vi "Keithley24XX_measure_snap.vi"() -> ()   [LabVIEW 2018]
uses:
  <instrlib>/Keithley 24XX/Public/Data/Read (Single Point).vi
  <instrlib>/Keithley 24XX/Keithley 24XX.lvlib
panel:
  out "output cluster":T1
  out "error out 2":errorcluster
  out "VISA resource name out":refnum<visa-resource-name>
  in  "error in (no error)":errorcluster
  in  "VISA resource name":refnum<visa-resource-name>
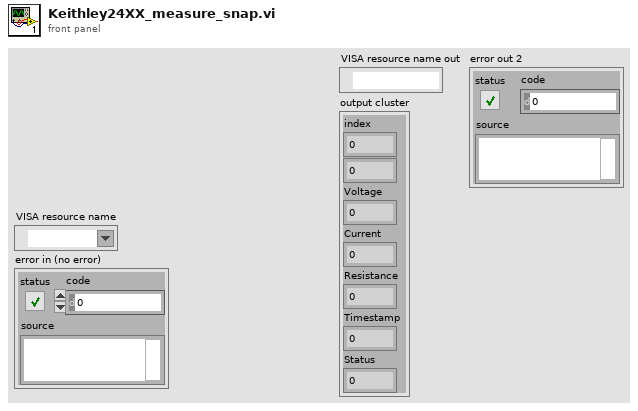
[diagram p1: front panel]
types:
  T1 = cluster{"index":i32, dbl, "Voltage":sgl, "Current":sgl, "Resistance":sgl, "Timestamp":sgl, "Status":sgl}
  T2 = cluster{"Source Mode":enum16{"Voltage", "Current"}, "Source Amplitude":dbl, "Timestamp":sgl, "Status":sgl, "Current":sgl, "Voltage":sgl, "Resistance":sgl}
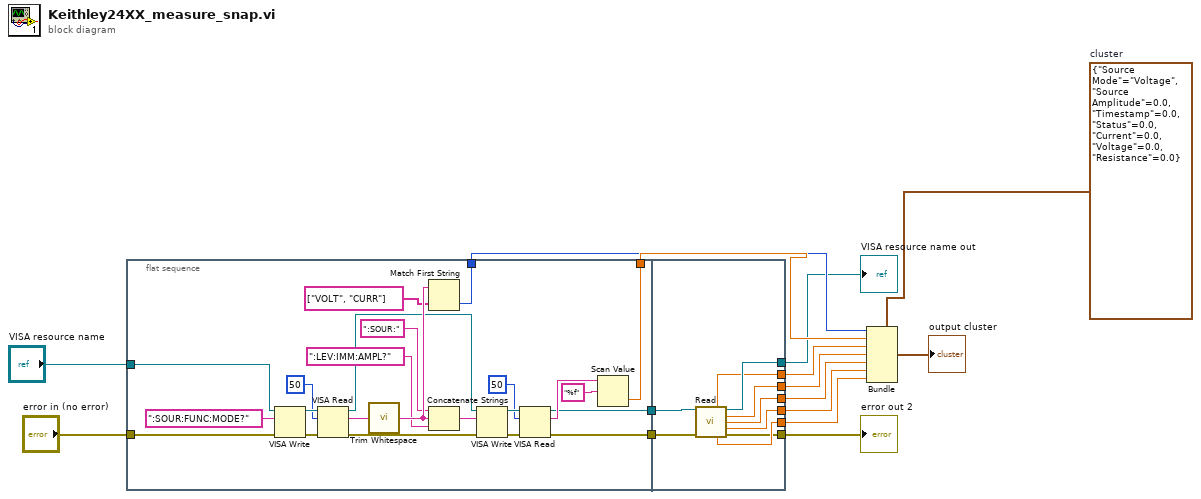
[diagram p0: block diagram]
diagram:
  w1 = T2 {"Source Mode"=enum."Voltage", "Source Amplitude"=0.0, "Timestamp"=0.0, "Status"=0.0, "Current"=0.0, "Voltage"=0.0, "Resistance"=0.0}  # cluster
  n1 = flat-sequence {
    tunnel: "VISA resource name" -> [w19]
    tunnel: "error in (no error)" -> [w18]
    tunnel: [w20] -> w13
    tunnel: [w21] -> w12
    tunnel: [w17] -> w11
    tunnel: [w16] -> w10
    tunnel: [w43] -> w3
    tunnel: [w44] -> w6
    tunnel: w11 -> [w47]
    tunnel: w10 -> [w46]
    tunnel: [w45] -> w9
    tunnel: [w42] -> w8
    tunnel: [w41] -> w7
    tunnel: [w40] -> w5
    tunnel: [w39] -> w4
    frame #0 {
      n2 = VISA Write(VISA resource name=w19, write buffer=":SOUR:FUNC:MODE?", error in (no error)=w18) -> (VISA resource name out=w30:refnum<visa-resource-name>, error out=w29:errorcluster)  [unwired: 1 out]
      n3 = VISA Read(VISA resource name=w30, byte count=u32 50, error in (no error)=w29) -> (VISA resource name out=w34:refnum<visa-resource-name>, read buffer=w37:string, error out=w33:errorcluster)  [unwired: 1 out]
      n4 = call <vilib>:"Trim Whitespace.vi"("string"=w37) -> ("trimmed string"=w38:string)  [unwired: 1 in]
      n5 = Match First String(2:string[] ["VOLT", "CURR"] ("string array"), 3:w38) -> (0:w21:i32)  [unwired: 1 out]
      n6 = Concatenate Strings(":SOUR:" ("string"), w38, ":LEV:IMM:AMPL?" ("string")) -> (w35:string)
      n7 = VISA Write(VISA resource name=w34, write buffer=w35, error in (no error)=w33) -> (VISA resource name out=w32:refnum<visa-resource-name>, error out=w31:errorcluster)  [unwired: 1 out]
      n8 = VISA Read(VISA resource name=w32, byte count=u32 50, error in (no error)=w31) -> (VISA resource name out=w17:refnum<visa-resource-name>, read buffer=w36:string, error out=w16:errorcluster)  [unwired: 1 out]
      n9 = Scan Value(string=w36, format string="%f") -> (value=w20:dbl)  [unwired: 1 in, 1 out]
    }
    frame #1 {
      n10 = call-poly <instrlib>:"Read.vi"("VISA resource name"=w47, "error in (no error)"=w46) -> ("Voltage"=w41:sgl, "VISA resource name out"=w45:refnum<visa-resource-name>, "Current"=w44:sgl, "Resistance"=w40:sgl, "Timestamp"=w39:sgl, "Status"=w43:sgl, "error out"=w42:errorcluster)  [unwired: 7 in]
    }
  }
  n11 = Bundle(cluster=w1, "Source Mode"=w12, "Source Amplitude"=w13, "Timestamp"=w7, "Status"=w6, "Current"=w5, "Voltage"=w4, "Resistance"=w3) -> (→"output cluster":T2)
  "VISA resource name out" <- w9
  "error out 2" <- w8
